vi "Project 7.vi"() -> ()   [LabVIEW 2017]
uses:
  <vilib>/NI/Modbus Library/API/Wrapper/Create TCP Master.vi
  <vilib>/NI/Modbus Library/API/Master/Modbus Master.lvclass
  <vilib>/NI/Modbus Library/API/Wrapper/API Main.lvlib
panel:
  out "Pass1":dbl
  out "Fail1":dbl
  out "total 1":dbl
  out "error out 10":errorcluster
  out "error out 9":errorcluster
  out "error out 8":errorcluster
  out "error out 7":errorcluster
  out "date/time string":string
  out "In Range?":bool
  out "error out 6":errorcluster
  out "error out 5":errorcluster
  out "Downtime 2":dbl
  out "Downtime beg":dbl caption="Elapsed Time (s)"
  out "current time":timestamp
  out "OEEc":dbl
  out "Qualityc":dbl
  out "Performancec":dbl
  out "Availabilityc":dbl
  out "Total Time":dbl caption="Elapsed Time (s)"
  out "Downtime":dbl caption="Elapsed Time (s)"
  out "Plot4":dbl=1000000.0
  out "Plot2":dbl=1000000.0
  out "Shift":string
  out "From":string
  out "TO":string
  out "OEE":dbl(knob) scale=0.0..100.0 scale format="%^_2g"
  out "Availability":dbl(knob) scale=0.0..100.0 scale format="%^_2g"
  out "Performance":dbl(knob) scale=0.0..100.0 scale format="%^_2g"
  out "Quality":dbl(knob) scale=0.0..100.0 scale format="%^_2g"
  out "error out":errorcluster
  out "x != y?":bool
  out "Fail":dbl
  out "Pass":dbl
  out "Total":dbl
  out "Waveform Chart 2":waveform(dbl)[](graph)
  out "register values":u16[](array[numeric])
  in  "address":string
  in  "port (502)":u16=502
  in  "error in":errorcluster
  # "Varroc"
  # "VEL III"
  # "SHIFT:"
  # "Excellence"
  # "COUNT"
  # "TIME"
  # "Total"
  # "Correct"
  # "Defective"
  # "DEFECTIVE"
  # "TOTAL"
  # "CORRECT"
  # "OEE"
  # "QUALITY"
  # "PERFORMANCE"
  # "AVAILABILITY"
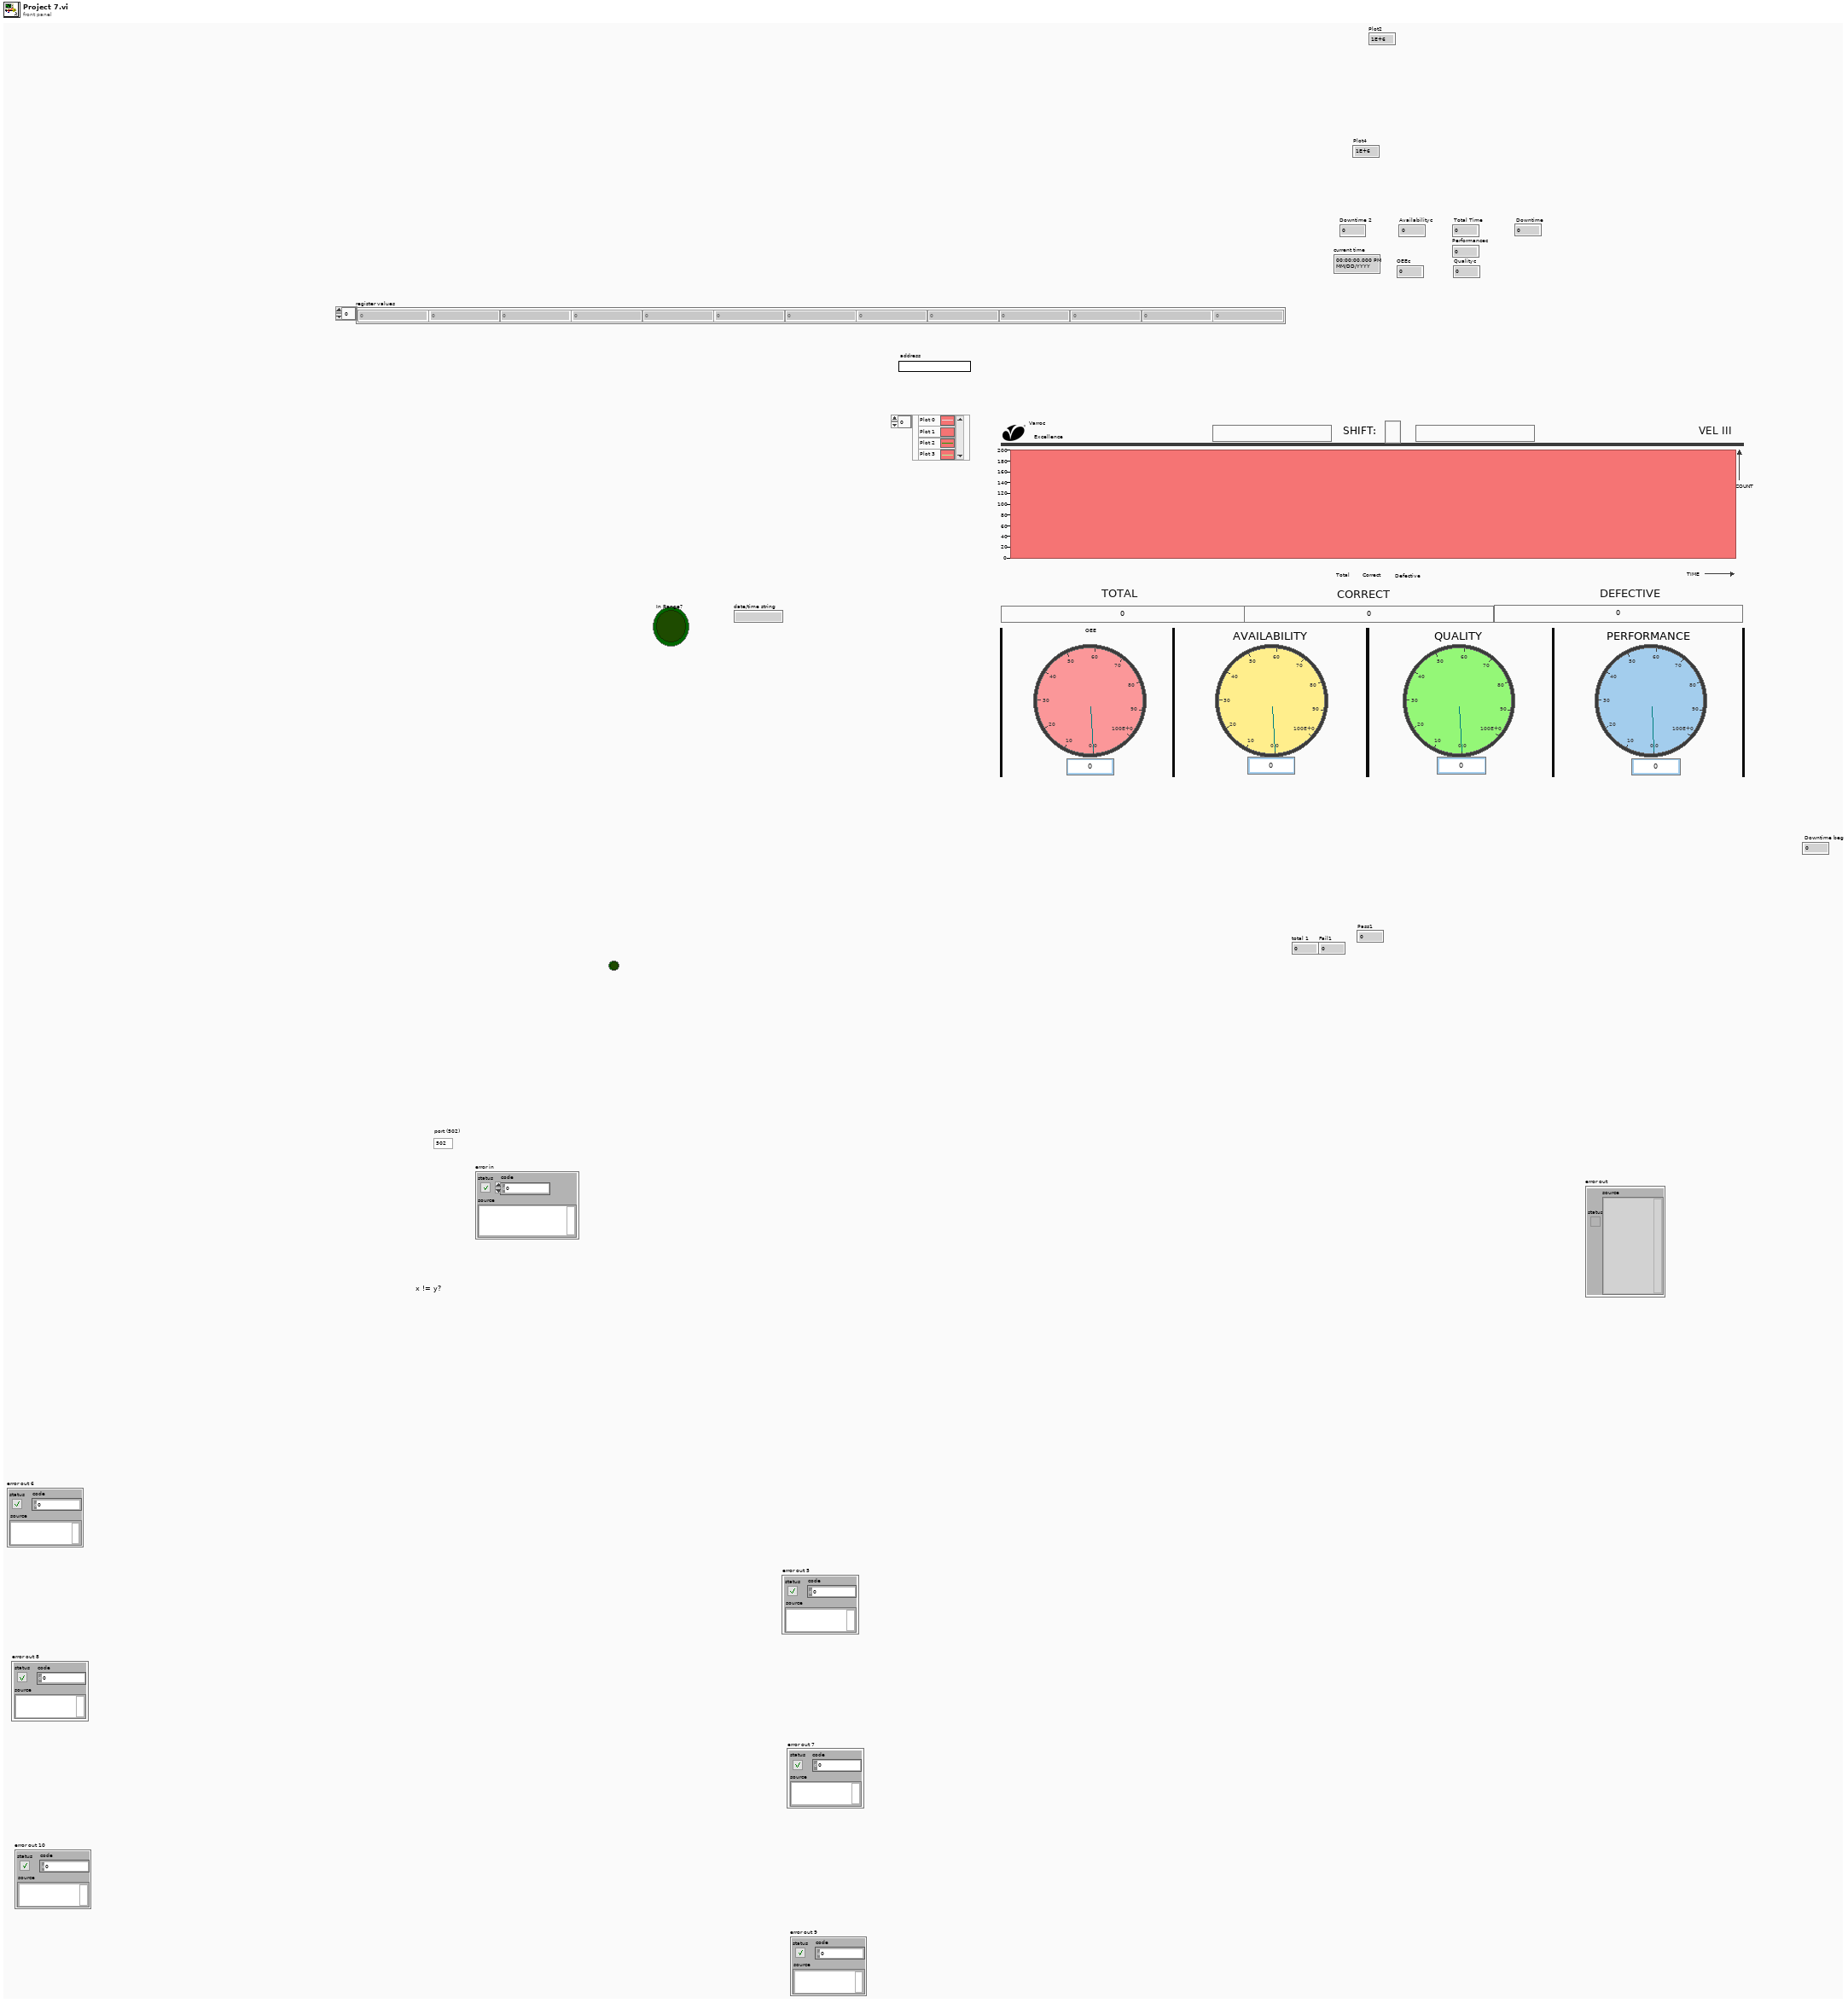
[diagram p1: front panel]
types:
  T1 = cluster{waveform(dbl), waveform(dbl), waveform(dbl), waveform(dbl)}
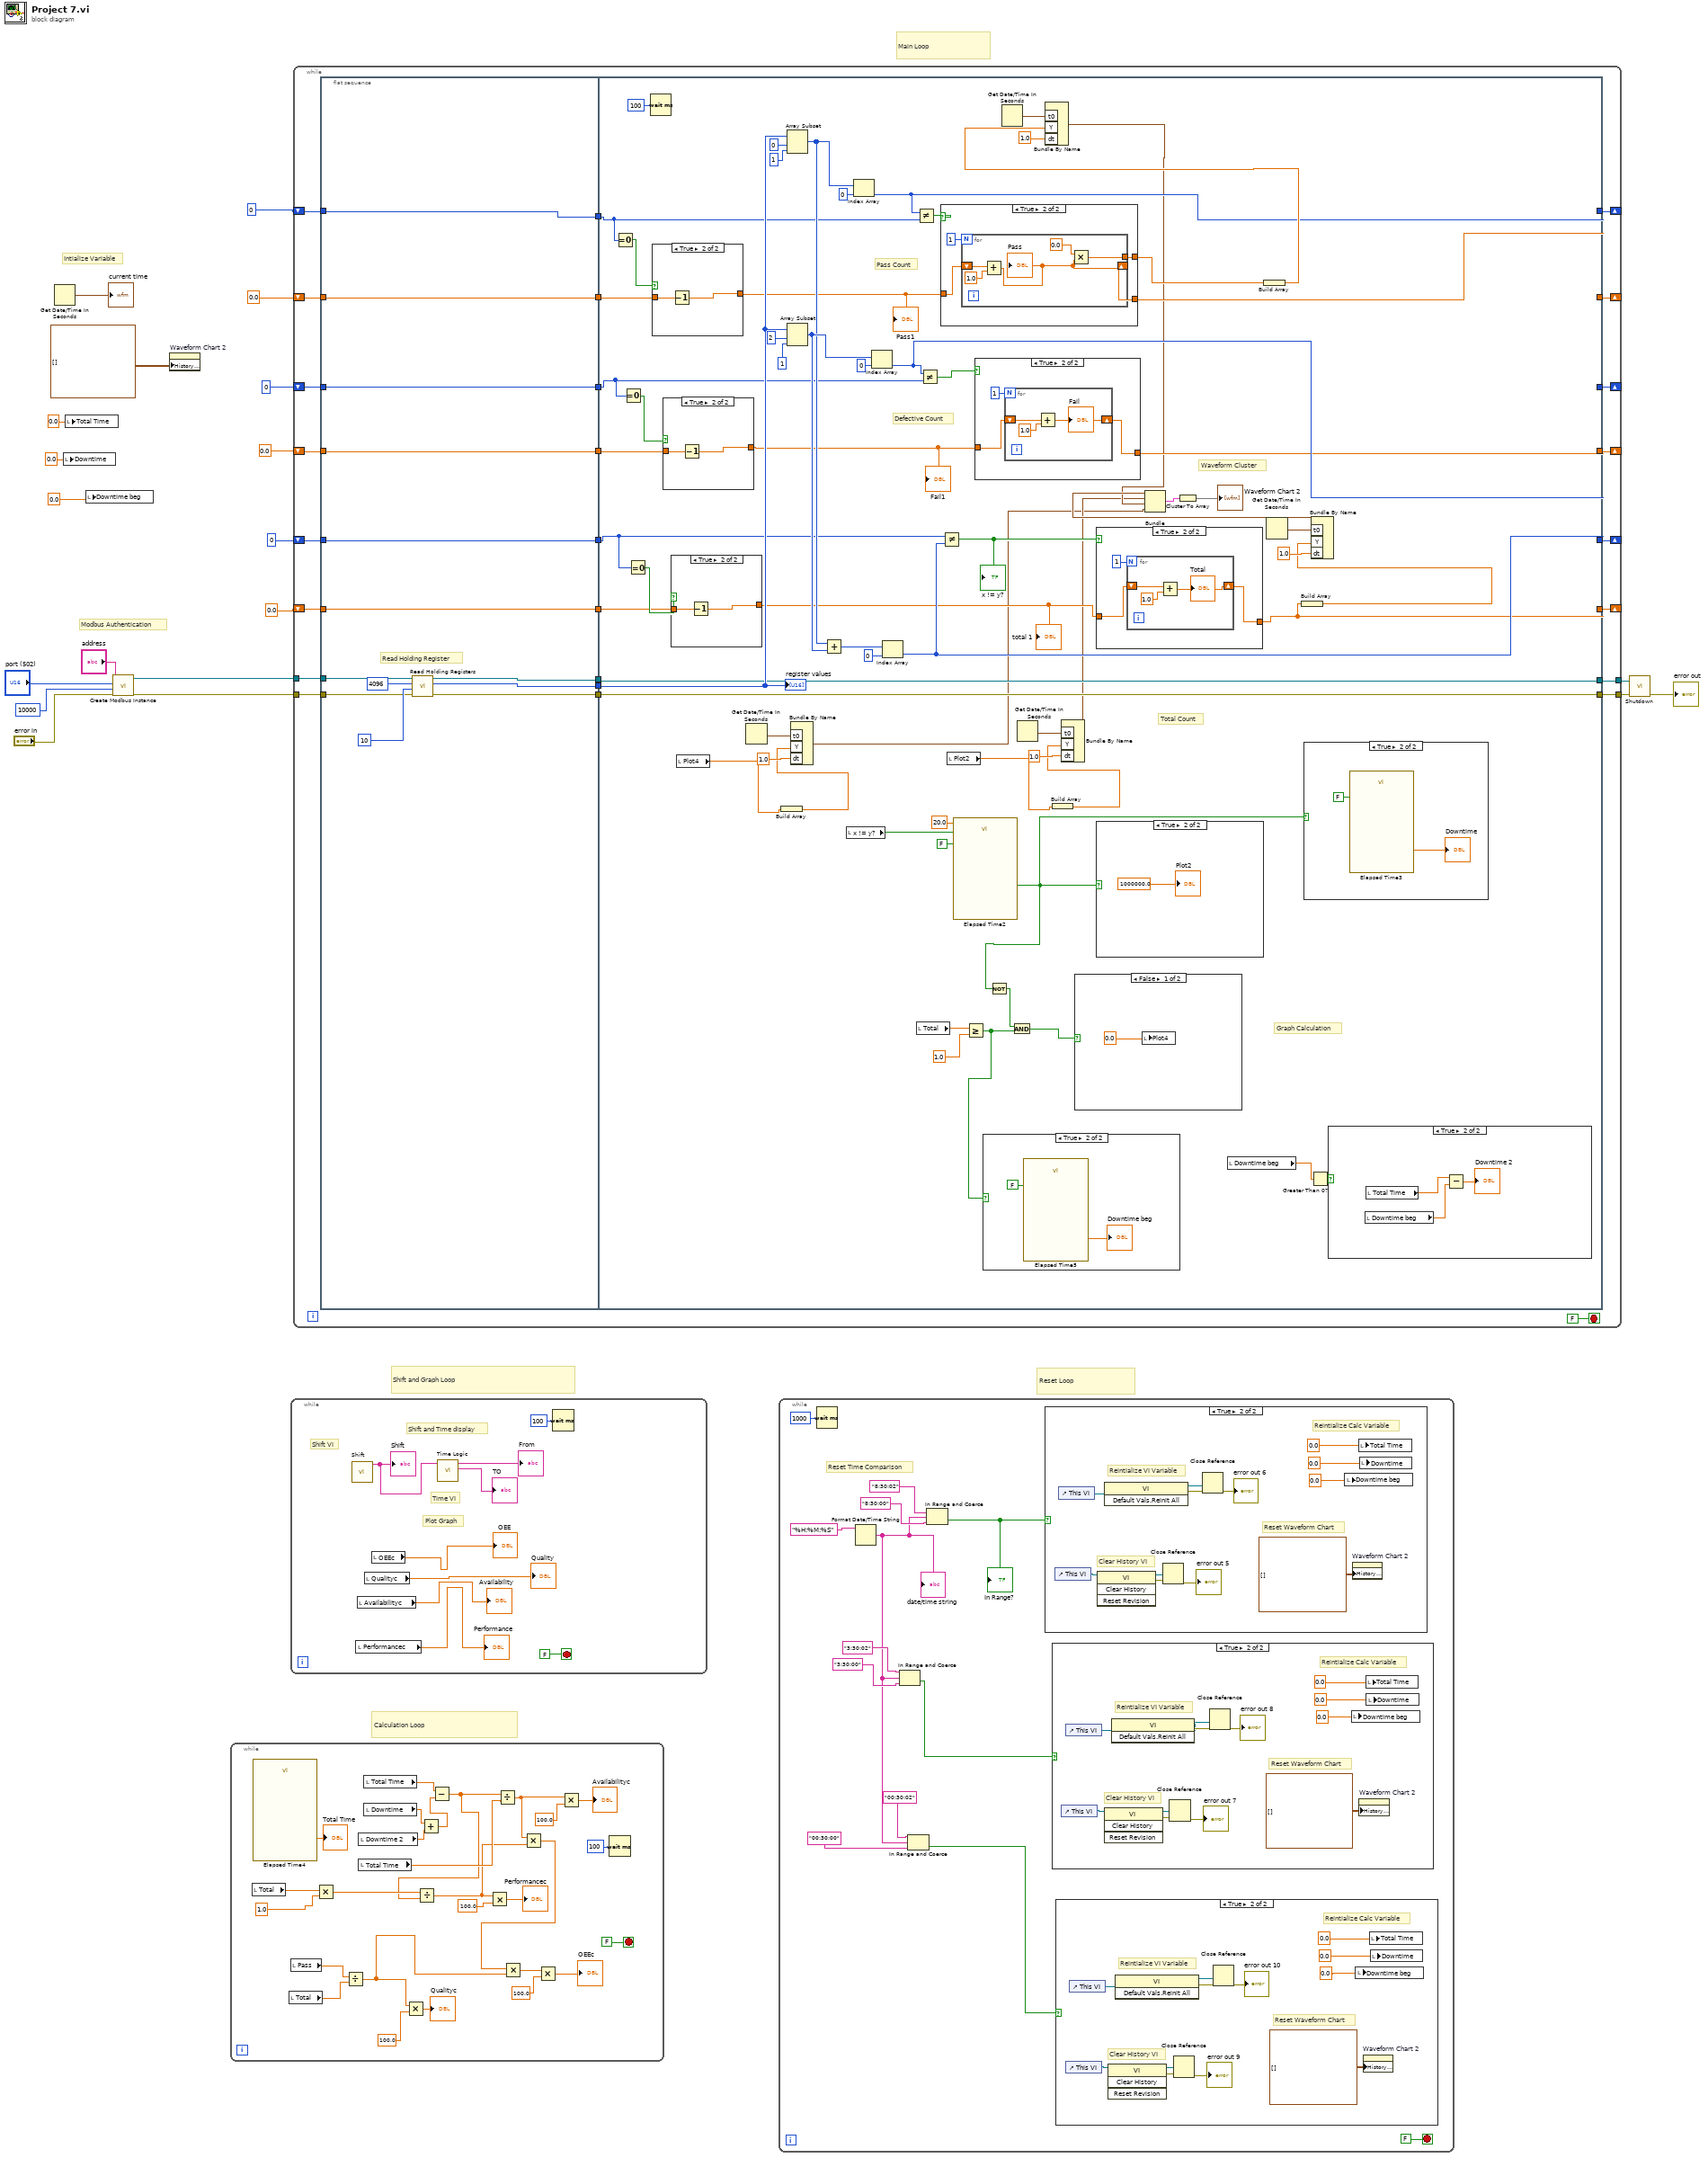
[diagram p0: block diagram]
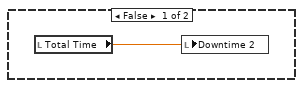
[diagram p5: hidden frame]
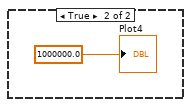
[diagram p8: hidden frame]
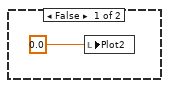
[diagram p9: hidden frame]
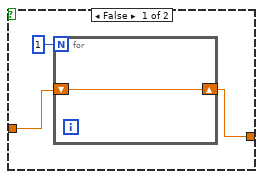
[diagram p13: hidden frame]
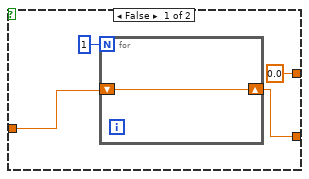
[diagram p14: hidden frame]
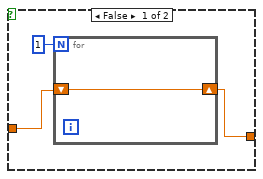
[diagram p15: hidden frame]
diagram:
  # "Main Loop"
  # "Intialize Variable"
  # "Modbus Authentication"
  # "Calculation Loop"
  # "Shift and Graph Loop"
  # "Reset Loop"
  n1 = Get Date/Time In Seconds() -> (seconds since 1Jan1904=→"current time":timestamp)
  n2 = local write "Downtime"(0.0 ("Downtime")) -> ()
  n3 = local write "Total Time"(0.0 ("Total Time")) -> ()
  n4 = local write "Downtime beg"(0.0 ("Downtime beg")) -> ()
  n5 = call-poly <vilib>:"Create Modbus Instance.vi"("error in"="error in", "connect timeout ms"=10000, "port (502)"="port (502)", "address"="address") -> ("error out"=w16:errorcluster, "TCP master instance"=w15:refnum<class "Modbus Master.lvclass">)  [unwired: 6 in]
  n6 = property on="Waveform Chart 2" class="WFChart (strict)"("History Data"=waveform(u32)[][] []) -> ()  [unwired: 2 in, 2 out]
  n7 = while {
    stop <- FALSE stop-if-true
    n8 = local read "Total"() -> (w43:dbl)
    n9 = call "Elapsed Time4"() -> ("Elapsed Time (s)"=→"Total Time":dbl)  [unwired: 12 in, 7 out]
    n10 = local read "Total"() -> (w39:dbl)
    n11 = local read "Pass"() -> (w40:dbl)
    n12 = Multiply(x=w43, y=1.0) -> (x*y=w41:dbl)
    n13 = Divide(x=w40, y=w39) -> (x/y=w29:dbl)
    n14 = local read "Downtime 2"() -> (w24:dbl)
    n15 = local read "Total Time"() -> (w44:dbl)
    n16 = local read "Total Time"() -> (w45:dbl)
    n17 = local read "Downtime"() -> (w23:dbl)
    n18 = Multiply(x=w29, y=100.0) -> (x*y=→"Qualityc":dbl)
    n19 = Add(x=w23, y=w24) -> (x+y=w22:dbl)
    n20 = Subtract(x=w45, y=w22) -> (x-y=w25:dbl)
    n21 = Divide(x=w41, y=w25) -> (x/y=w34:dbl)
    n22 = Multiply(x=w34, y=100.0) -> (x*y=→"Performancec":dbl)
    n23 = Divide(x=w25, y=w44) -> (x/y=w26:dbl)
    n24 = Multiply(x=w26, y=w34) -> (x*y=w38:dbl)
    n25 = Multiply(x=w38, y=w29) -> (x*y=w37:dbl)
    n26 = Multiply(x=w37, y=100.0) -> (x*y=→"OEEc":dbl)
    n27 = Multiply(x=w26, y=100.0) -> (x*y=→"Availabilityc":dbl)
    n28 = Wait (ms)(milliseconds to wait=u32 100) -> ()  [unwired: 1 out]
  }
  n29 = while {
    stop <- FALSE stop-if-true
    # "Time VI"
    # "Shift VI"
    # "Shift and Time display"
    # "Plot Graph"
    n30 = call "Shift.vi"() -> ("Shift"=w55:string)  [unwired: 10 in]
    "Shift" <- w55
    n31 = local read "Performancec"() -> (→"Performance":dbl)
    n32 = local read "Availabilityc"() -> (→"Availability":dbl)
    n33 = local read "Qualityc"() -> (→"Quality":dbl)
    n34 = local read "OEEc"() -> (→"OEE":dbl)
    n35 = call "Time Logic.vi"("Shift"=w55) -> ("TO"=→"TO":string, "From"=→"From":string)  [unwired: 9 in]
    n36 = Wait (ms)(milliseconds to wait=u32 100) -> ()  [unwired: 1 out]
  }
  n37 = while {
    tunnel: w16 -> [w81]
    tunnel: w15 -> [w82]
    tunnel: [w77] -> w13
    tunnel: [w76] -> w12
    shift-right: [w58] -> _
    shift-left: 0 ("index") -> [w74]
    shift-right: [w63] -> _
    shift-left: 0.0 ("y") -> [w72]
    shift-right: [w62] -> _
    shift-left: 0 ("index") -> [w70]
    shift-right: [w61] -> _
    shift-left: 0.0 ("y") -> [w68]
    shift-right: [w60] -> _
    shift-left: 0 ("index") -> [w66]
    shift-right: [w59] -> _
    shift-left: 0.0 ("y") -> [w64]
    stop <- FALSE stop-if-true
    n38 = flat-sequence {
      tunnel: w82 -> [w93]
      tunnel: w81 -> [w92]
      tunnel: [w91] -> w80
      tunnel: [w90] -> w79
      tunnel: [w89] -> w78
      tunnel: [w88] -> w75
      tunnel: w74 -> [w88]
      tunnel: [w87] -> w73
      tunnel: w72 -> [w87]
      tunnel: [w86] -> w71
      tunnel: w70 -> [w86]
      tunnel: [w85] -> w69
      tunnel: w68 -> [w85]
      tunnel: [w84] -> w67
      tunnel: w66 -> [w84]
      tunnel: [w83] -> w65
      tunnel: w64 -> [w83]
      tunnel: w80 -> [w139]
      tunnel: w79 -> [w138]
      tunnel: w78 -> [w137]
      tunnel: [w138] -> w77
      tunnel: [w137] -> w76
      tunnel: w75 -> [w130]
      tunnel: w73 -> [w128]
      tunnel: w71 -> [w123]
      tunnel: w69 -> [w125]
      tunnel: w67 -> [w120]
      tunnel: w65 -> [w121]
      tunnel: [w135] -> w63
      tunnel: [w136] -> w58
      tunnel: [w134] -> w62
      tunnel: [w133] -> w61
      tunnel: [w132] -> w60
      tunnel: [w131] -> w59
      frame #0 {
        # "Read Holding Register"
        n39 = call-dynamic "Read Holding Registers.vi"("error in"=w92, "number of inputs"=u16 10, "starting address"=u16 4096, "Modbus master in"=w93) -> ("error out"=w89:errorcluster, "register values"=w91:u16[], "Modbus master out"=w90:refnum<class "Modbus Master.lvclass">)  [unwired: 5 in]
      }
      frame #1 {
        # "Graph Calculation"
        # "Pass Count"
        # "Defective Count"
        # "Total Count"
        # "Waveform Cluster"
        n40 = Equal To 0?(x=w130) -> (x = 0?=w129:bool)
        n41 = Equal To 0?(x=w123) -> (x = 0?=w126:bool)
        n42 = Equal To 0?(x=w120) -> (x = 0?=w122:bool)
        n43 = Wait (ms)(milliseconds to wait=u32 100) -> ()  [unwired: 1 out]
        n44 = case shown="True" w129 {
          tunnel: w128 -> [w181 w183]
          tunnel: [w181 w182] -> w127
          frame False {
          }
          frame True {
            n45 = Decrement(x=w183) -> (x-1=w182:dbl)
          }
        }
        "Pass1" <- w127
        n46 = case shown="True" w126 {
          tunnel: w125 -> [w178 w180]
          tunnel: [w178 w179] -> w124
          frame False {
          }
          frame True {
            n47 = Decrement(x=w180) -> (x-1=w179:dbl)
          }
        }
        "Fail1" <- w124
        n48 = case shown="True" w122 {
          tunnel: w121 -> [w175 w177]
          tunnel: [w175 w176] -> w119
          frame False {
          }
          frame True {
            n49 = Decrement(x=w177) -> (x-1=w176:dbl)
          }
        }
        "total 1" <- w119
        n50 = local read "Plot4"() -> (w102:dbl)
        n51 = Get Date/Time In Seconds() -> (seconds since 1Jan1904=w104:timestamp)
        n52 = Build Array(w102) -> (w103:dbl[])
        n53 = Array Subset(array=w139, index=0, length=1) -> (w146:u16[])
        n54 = Array Subset(array=w139, index=2, length=1) -> (w154:u16[])
        n55 = Bundle By Name("t0"=w104, "Y"=w103, "dt"=1.0) -> (w101:waveform(dbl))  [unwired: 1 in]
        n56 = Add(x=w146, y=w154) -> (x+y=w152:u16[])
        n57 = local read "x != y?"() -> (w117:bool)
        n58 = Index Array(array=w146, index=0) -> (element=w136:u16)
        n59 = Index Array(array=w154, index=0) -> (element=w134:u16)
        n60 = Index Array(array=w152, index=0) -> (element=w132:u16)
        n61 = Not Equal?(x=w136, y=w130) -> (x != y?=w145:bool)
        n62 = local read "Total"() -> (w109:dbl)
        n63 = Not Equal?(x=w134, y=w123) -> (x != y?=w144:bool)
        n64 = case shown="True" w145 {
          tunnel: w127 -> [w196 w201]
          tunnel: [w195 w200] -> w135
          tunnel: [0.0 w199] -> w140
          frame False {
            n65 = for {
              N: 1 -> [_]
              shift-right: [w198] -> w195
              shift-left: w196 -> [w198]
            }
          }
          frame True {
            n66 = for {
              N: 1 -> [_]
              shift-right: [w203] -> w200
              shift-left: w201 -> [w207]
              tunnel: [w205] -> w199
              n67 = Add(x=w207, y=1.0) -> (x+y=w203:dbl)
              "Pass" <- w203
              n68 = Multiply(x=0.0, y=w203) -> (x*y=w205:dbl)
            }
          }
        }
        n69 = Not Equal?(x=w120, y=w132) -> (x != y?=w143:bool)
        "x != y?" <- w143
        n70 = local read "Plot2"() -> (w112:dbl)
        n71 = call "Elapsed Time2"("Time Target (s)"=20.0, "Reset"=w117, "Auto Reset"=FALSE) -> ("Time has Elapsed"=w99:bool)  [unwired: 9 in, 7 out]
        n72 = Greater Or Equal?(x=w109, y=1.0) -> (x >= y?=w98:bool)
        n73 = case shown="True" w144 {
          tunnel: w124 -> [w185 w189]
          tunnel: [w184 w188] -> w133
          frame False {
            n74 = for {
              N: 1 -> [_]
              shift-right: [w187] -> w184
              shift-left: w185 -> [w187]
            }
          }
          frame True {
            n75 = for {
              N: 1 -> [_]
              shift-right: [w191] -> w188
              shift-left: w189 -> [w193]
              n76 = Add(x=w193, y=1.0) -> (x+y=w191:dbl)
              "Fail" <- w191
            }
          }
        }
        n77 = case shown="True" w98 {
          frame False {
          }
          frame True {
            n78 = call "Elapsed Time5"("Auto Reset"=FALSE) -> ("Elapsed Time (s)"=→"Downtime beg":dbl)  [unwired: 11 in, 7 out]
          }
        }
        n79 = Not(x=w99) -> (.not. x?=w106:bool)
        n80 = Get Date/Time In Seconds() -> (seconds since 1Jan1904=w159:timestamp)
        n81 = And(x=w106, y=w98) -> (x .and. y?=w107:bool)
        n82 = Get Date/Time In Seconds() -> (seconds since 1Jan1904=w114:timestamp)
        n83 = Build Array(w112) -> (w113:dbl[])
        n84 = Bundle By Name("t0"=w114, "Y"=w113, "dt"=1.0) -> (w110:waveform(dbl))  [unwired: 1 in]
        n85 = case shown="False" w107 {
          frame False {
            n86 = local write "Plot4"(0.0 ("Time Target (s)")) -> ()
          }
          frame True {
            "Plot4" <- 1000000.0 ("dt")
          }
        }
        n87 = case shown="True" w143 {
          tunnel: w119 -> [w209 w213]
          tunnel: [w208 w212] -> w131
          frame False {
            n88 = for {
              N: 1 -> [_]
              shift-right: [w211] -> w208
              shift-left: w209 -> [w211]
            }
          }
          frame True {
            n89 = for {
              N: 1 -> [_]
              shift-right: [w215] -> w212
              shift-left: w213 -> [w217]
              n90 = Add(x=w217, y=1.0) -> (x+y=w215:dbl)
              "Total" <- w215
            }
          }
        }
        n91 = case shown="True" w99 {
          frame False {
            n92 = local write "Plot2"(0.0 ("Time Target (s)")) -> ()
          }
          frame True {
            "Plot2" <- 1000000.0 ("dt")
          }
        }
        n93 = local read "Downtime beg"() -> (w96:dbl)
        n94 = Build Array(w140) -> (w142:dbl[])
        n95 = Bundle By Name("t0"=w159, "Y"=w142, "dt"=1.0) -> (w111:waveform(dbl))  [unwired: 1 in]
        n96 = Get Date/Time In Seconds() -> (seconds since 1Jan1904=w148:timestamp)
        n97 = Build Array(w131) -> (w141:dbl[])
        n98 = case shown="True" w99 {
          frame False {
          }
          frame True {
            n99 = call "Elapsed Time3"("Auto Reset"=FALSE) -> ("Elapsed Time (s)"=→"Downtime":dbl)  [unwired: 11 in, 7 out]
          }
        }
        n100 = Greater Than 0?(x=w96) -> (x > 0?=w97:bool)
        n101 = Bundle By Name("t0"=w148, "Y"=w141, "dt"=1.0) -> (w147:waveform(dbl))  [unwired: 1 in]
        n102 = Bundle(w147, w110, w111, w101) -> (w149:T1)  [unwired: 1 in]
        n103 = Cluster To Array(cluster=w149) -> (array=→"Waveform Chart 2":waveform(dbl)[])
        n104 = case shown="True" w97 {
          frame False {
            n105 = local read "Total Time"() -> (w163:dbl)
            n106 = local write "Downtime 2"(w163) -> ()
          }
          frame True {
            n107 = local read "Downtime beg"() -> (w164:dbl)
            n108 = local read "Total Time"() -> (w165:dbl)
            n109 = Subtract(x=w165, y=w164) -> (x-y=→"Downtime 2":dbl)
          }
        }
        "register values" <- w139
      }
    }
  }
  n110 = while {
    stop <- FALSE stop-if-true
    # "Reset Time Comparison"
    n111 = Wait (ms)(milliseconds to wait=u32 1000) -> ()  [unwired: 1 out]
    n112 = Format Date/Time String(time format string (%c)="%H:%M:%S") -> (date/time string=w222:string)  [unwired: 2 in]
    "date/time string" <- w222
    n113 = In Range and Coerce(upper limit="3:30:02" ("String"), x=w222, lower limit="3:30:00" ("String")) -> (In Range?=w219:bool)  [unwired: 1 out]
    n114 = In Range and Coerce(upper limit="00:30:02" ("String"), x=w222, lower limit="00:30:00" ("String")) -> (In Range?=w218:bool)  [unwired: 1 out]
    n115 = In Range and Coerce(upper limit="8:30:02" ("String"), x=w222, lower limit="8:30:00" ("String")) -> (In Range?=w220:bool)  [unwired: 1 out]
    "In Range?" <- w220
    n116 = case shown="True" w220 {
      frame False {
      }
      frame True {
        # "Reintialize VI Variable"
        # "Clear History VI"
        # "Reintialize Calc Variable"
        # "Reset Waveform Chart"
        n117 = control-ref of="This VI"() -> (w261:refnum<vi>)
        n118 = control-ref of="This VI"() -> (w263:refnum<vi>)
        n119 = invoke class="VI" method="Clear History"(reference=w261) -> (reference out=w259:refnum<vi>, error out=w258:errorcluster)  [unwired: 3 in, 2 out]
        n120 = invoke class="VI" method="Default Vals.Reinit All"(reference=w263) -> (reference out=w265:refnum<vi>, error out=w266:errorcluster)  [unwired: 2 in, 1 out]
        n121 = Close Reference(reference=w259, error in (no error)=w258) -> (error out=→"error out 5":errorcluster)
        n122 = Close Reference(reference=w265, error in (no error)=w266) -> (error out=→"error out 6":errorcluster)
        n123 = local write "Downtime beg"(0.0 ("Downtime beg")) -> ()
        n124 = property on="Waveform Chart 2" class="WFChart (strict)"("History Data"=waveform(u32)[][] []) -> ()  [unwired: 2 in, 2 out]
        n125 = local write "Total Time"(0.0 ("Total Time")) -> ()
        n126 = local write "Downtime"(0.0 ("Downtime")) -> ()
      }
    }
    n127 = case shown="True" w219 {
      frame False {
      }
      frame True {
        # "Reintialize VI Variable"
        # "Clear History VI"
        # "Reintialize Calc Variable"
        # "Reset Waveform Chart"
        n128 = control-ref of="This VI"() -> (w249:refnum<vi>)
        n129 = control-ref of="This VI"() -> (w251:refnum<vi>)
        n130 = invoke class="VI" method="Clear History"(reference=w249) -> (reference out=w247:refnum<vi>, error out=w246:errorcluster)  [unwired: 3 in, 2 out]
        n131 = invoke class="VI" method="Default Vals.Reinit All"(reference=w251) -> (reference out=w253:refnum<vi>, error out=w254:errorcluster)  [unwired: 2 in, 1 out]
        n132 = Close Reference(reference=w247, error in (no error)=w246) -> (error out=→"error out 7":errorcluster)
        n133 = Close Reference(reference=w253, error in (no error)=w254) -> (error out=→"error out 8":errorcluster)
        n134 = local write "Downtime beg"(0.0 ("Downtime beg")) -> ()
        n135 = property on="Waveform Chart 2" class="WFChart (strict)"("History Data"=waveform(u32)[][] []) -> ()  [unwired: 2 in, 2 out]
        n136 = local write "Total Time"(0.0 ("Total Time")) -> ()
        n137 = local write "Downtime"(0.0 ("Downtime")) -> ()
      }
    }
    n138 = case shown="True" w218 {
      frame False {
      }
      frame True {
        # "Reintialize VI Variable"
        # "Clear History VI"
        # "Reintialize Calc Variable"
        # "Reset Waveform Chart"
        n139 = control-ref of="This VI"() -> (w237:refnum<vi>)
        n140 = control-ref of="This VI"() -> (w239:refnum<vi>)
        n141 = invoke class="VI" method="Clear History"(reference=w237) -> (reference out=w235:refnum<vi>, error out=w234:errorcluster)  [unwired: 3 in, 2 out]
        n142 = invoke class="VI" method="Default Vals.Reinit All"(reference=w239) -> (reference out=w241:refnum<vi>, error out=w242:errorcluster)  [unwired: 2 in, 1 out]
        n143 = Close Reference(reference=w235, error in (no error)=w234) -> (error out=→"error out 9":errorcluster)
        n144 = Close Reference(reference=w241, error in (no error)=w242) -> (error out=→"error out 10":errorcluster)
        n145 = local write "Downtime beg"(0.0 ("Downtime beg")) -> ()
        n146 = property on="Waveform Chart 2" class="WFChart (strict)"("History Data"=waveform(u32)[][] []) -> ()  [unwired: 2 in, 2 out]
        n147 = local write "Total Time"(0.0 ("Total Time")) -> ()
        n148 = local write "Downtime"(0.0 ("Downtime")) -> ()
      }
    }
  }
  n149 = call-dynamic "Shutdown.vi"("error in"=w12, "Modbus master in"=w13) -> ("error out"=→"error out":errorcluster)  [unwired: 9 in]
